vi "Initialize.vi"(8 "error in (no error)":errorcluster, 11 "Core Thread User Interface in":refnum<class "Core Thread User Interface.lvclass">) -> (0 "error out":errorcluster, 3 "Core Thread User Interface out":refnum<class "Core Thread User Interface.lvclass">)   [LabVIEW 2017, in "DSF Core.lvlib" / "Core Thread User Interface.lvclass"]
uses:
  Core Thread User Interface.lvclass
  C:/Git/DSF/Core/Classes/User Interface/User Interface.lvclass
  Configuration/Core/Thread/Thread Configuration.lvclass
  C:/Git/DSF/Core/Classes/Configuration/Configuration.lvclass
  User Interface.lvclass
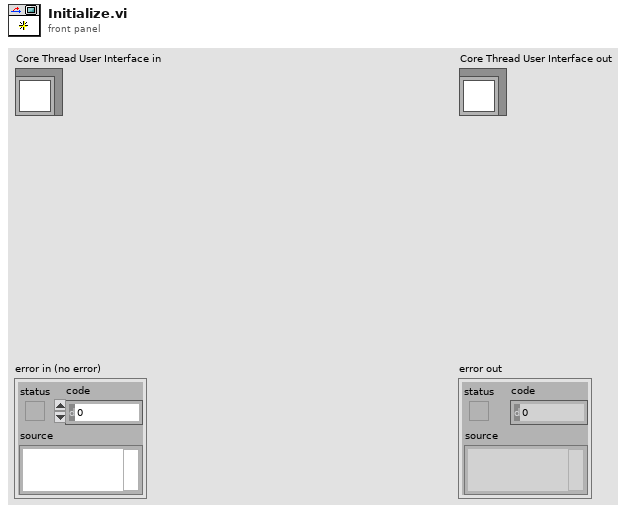
[diagram p1: front panel]
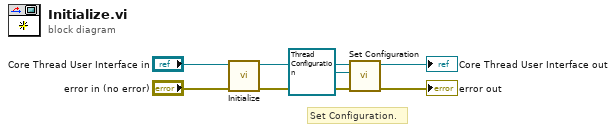
[diagram p0: block diagram]
diagram:
  # "Set Configuration."
  n1 = call-parent "Initialize.vi"("error in (no error)"="error in (no error)", "User Interface in"="Core Thread User Interface in") -> ("error out"=w1:errorcluster, "User Interface out"=w2:refnum<class "Core Thread User Interface.lvclass">)  [unwired: 8 in]
  n2 = call "Set Configuration.vi"("error in (no error)"=w1, "configuration"=refnum<class "Thread Configuration.lvclass"> refnum ("DSF Core.lvlib:Thread Configuration.lvclass"), "User Interface in"=w2) -> ("error out"=→"error out":errorcluster, "User Interface out"=→"Core Thread User Interface out":refnum<class "Core Thread User Interface.lvclass">)  [unwired: 7 in]
